vi "catalog.create_dataset.request.vi"(8 "error in":errorcluster, 11 "name":string) -> (0 "error out":errorcluster, 3 "request":string)   [LabVIEW 2020, in "Nominal Client.lvclass"]
uses:
  Nominal Client.lvclass
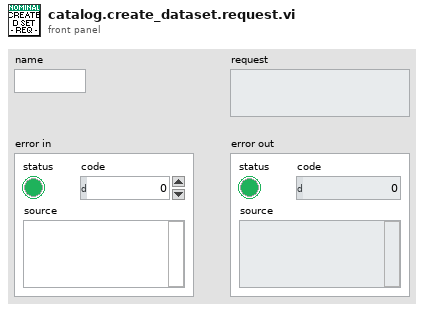
[diagram p1: front panel]
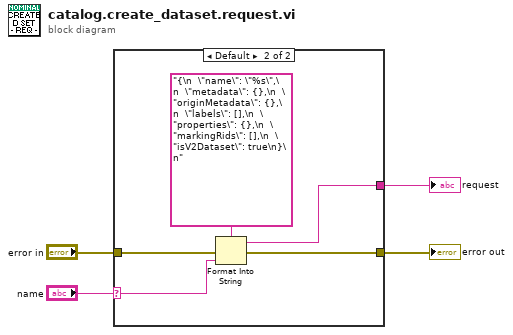
[diagram p0: block diagram]
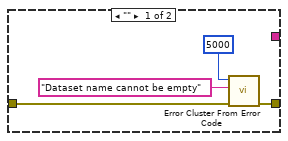
[diagram p2: hidden frame]
diagram:
  n1 = case shown="Default" "name" {
    selector: "name" -> [_ w12]
    tunnel: "error in" -> [w8 w11]
    tunnel: [_ w10] -> w2
    tunnel: [w7 w9] -> w1
    frame "" {
      n2 = call <vilib>:"Error Cluster From Error Code.vi"("error in (no error)"=w8, "error message (\"\")"="Dataset name cannot be empty" ("error message (\"\")"), "error code (0)"=5000) -> ("error out"=w7:errorcluster)  [unwired: 6 in]
    }
    frame Default {
      n3 = Format Into String(format string="{\n  \"name\": \"%s\",\n  \"metadata\": {},\n  \"originMetadata\": {},\n  \"labels\": [],\n  \"properties\": {},\n  \"markingRids\": [],\n  \"isV2Dataset\": true\n}\n" ("Request body"), error in=w11, w12) -> (resulting string=w10:string, error out=w9:errorcluster)  [unwired: 1 in]
    }
  }
  "error out" <- w1
  "request" <- w2
